vi "Auth Method.vi"(11 "WampCraaAuthenticator in":refnum<class "WampCraAuthenticator.lvclass">) -> (2 "Authmethod":string, 3 "WampCraaAuthenticator out":refnum<class "WampCraAuthenticator.lvclass">)   [LabVIEW 2020, in "wamplv.lvlib" / "WampCraAuthenticator.lvclass"]
uses:
  WampCraAuthenticator.lvclass
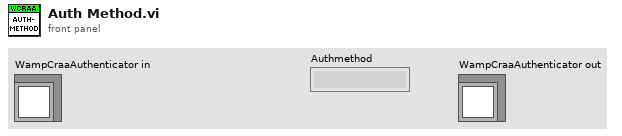
[diagram p1: front panel]
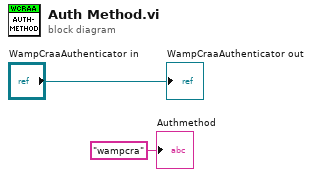
[diagram p0: block diagram]
diagram:
  "WampCraaAuthenticator out" <- "WampCraaAuthenticator in"
  "Authmethod" <- "wampcra" ("Authmethod")
